vi "Function.vi"(8 "error in (no error)":errorcluster, 10 "Value":sgl, 11 "Two Terminal in":refnum<class "Reciprocal_SGL.lvclass">) -> (0 "error out":errorcluster, 2 "Result":sgl, 3 "Two Terminal out":refnum<class "Reciprocal_SGL.lvclass">)   [LabVIEW 2021, in "Reciprocal_SGL.lvclass"]
uses:
  Reciprocal_SGL.lvclass
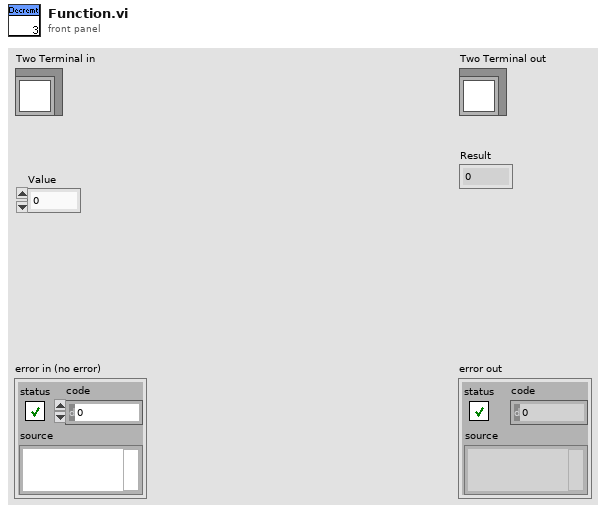
[diagram p1: front panel]
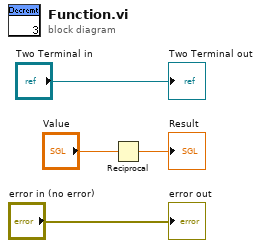
[diagram p0: block diagram]
diagram:
  n1 = Reciprocal(x="Value") -> (1/x=→"Result":sgl)
  "error out" <- "error in (no error)"
  "Two Terminal out" <- "Two Terminal in"
